vi "SumMajoritySelector.vi"(1 "On Sum\nOff Majority":bool, 6 "error in (no error)":errorcluster, 9 "connection ID":refnum<k5>) -> (0 "error out":errorcluster, 3 "connection ID out":refnum<k5>)   [LabVIEW 2012]
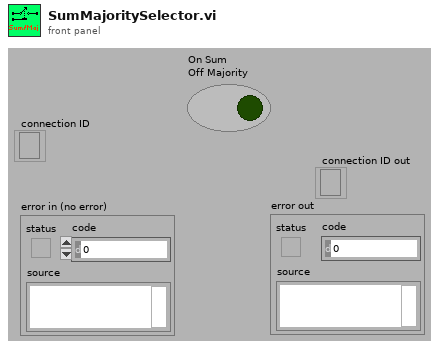
[diagram p1: front panel]
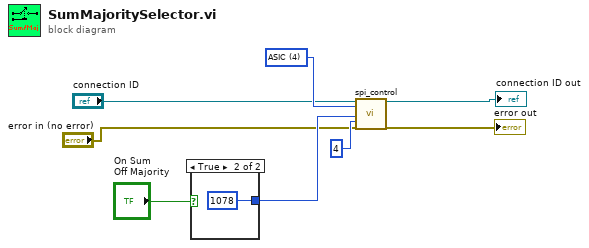
[diagram p0: block diagram]
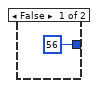
[diagram p2: hidden frame]
diagram:
  w8 = u16 4 items=["Attenuation", "Clipping", "Enable channel", "Delay line", "ASIC"] ("Device")
  n1 = case shown="True" "On Sum\nOff Majority" {
    tunnel: [56 ("Data") 1078 ("Data")] -> w6
    frame False {
    }
    frame True {
    }
  }
  n2 = call "spi_control.vi"("connection ID"="connection ID", "Device"=w8, "Data"=w6, "Register or channel"=4, "error in"="error in (no error)") -> ("connection ID out"=→"connection ID out":refnum<k5>, "error out 2"=→"error out":errorcluster)  [unwired: 7 in, 6 out]
